vi "TestConfig.vi"(8 "error in":errorcluster {"code" format="Error %.0f"}, 11 "MainFGV_data":T1) -> (0 "error out":errorcluster {"code" format="Error %.0f"}, 3 "MainFGV_data out":T1)   [LabVIEW 2016]
uses:
  StrainGauge/SG_data.ctl
  CurrentMeter/CM_data.ctl
  CurrentMeter/CM_SerialNumber.ctl
  MainFGV_data.ctl
  Log/log_mods.ctl
  Log/log_status.ctl
panel:
  in  "OK":bool
  in  "Cancelar":bool
  in  "OpenConfig":bool caption="Abrir\nconfiguração"
  in  "SaveConfig":bool caption="Salvar\nconfiguração"
  in  "CM_config":T2[](array[typedef])=[{"Serial"=enum."274124", "Coordenada X"=0.0, "Coordenada Y"=0.0, "ID"="CH 1", "active"=TRUE}, {"Serial"=enum."274125", "Coordenada X"=0.0, "Coordenada Y"=0.0, "ID"="CH 2", "active"=TRUE}, {"Serial"=enum."274126", "Coordenada X"=0.0, "Coordenada Y"=0.0, "ID"="CH 3", "active"=TRUE}, {"Serial"=enum."274127", "Coordenada X"=0.0, "Coordenada Y"=0.0, "ID"="CH 4", "active"=TRUE}, {"Serial"=enum."274128", "Coordenada X"=0.0, "Coordenada Y"=0.0, "ID"="CH 5", "active"=TRUE}]
  in  "SG_config":T4[](array[typedef])=[{"ID"="CH 1", "Sensibilidade"=2.0, "Descrição"="Extensômetro na grade", "active"=TRUE}, {"ID"="CH 2", "Sensibilidade"=2.0, "Descrição"="Extensômetro na grade", "active"=TRUE}, {"ID"="CH 3", "Sensibilidade"=2.0, "Descrição"="Extensômetro na grade", "active"=TRUE}, {"ID"="CH 4", "Sensibilidade"=2.0, "Descrição"="Extensômetro na grade", "active"=TRUE}, {"ID"="CH 5", "Sensibilidade"=2.0, "Descrição"="Extensômetro na grade", "active"=TRUE}, {"ID"="CH 6", "Sensibilidade"=2.0, "Descrição"="Extensômetro na grade", "active"=TRUE}, {"ID"="CH 7", "Sensibilidade"=2.0, "Descrição"="Extensômetro na grade", "active"=TRUE}, {"ID"="CH 8", "Sensibilidade"=2.0, "Descrição"="Extensômetro na grade", "active"=TRUE}, {"ID"="CH 9", "Sensibilidade"=2.0, "Descrição"="Extensômetro na grade", "active"=TRUE}, {"ID"="CH 10", "Sensibilidade"=2.0, "Descrição"="Extensômetro na grade", "active"=TRUE}, {"ID"="CH 11", "Sensibilidade"=2.0, "Descrição"="Extensômetro na grade", "active"=TRUE}, {"ID"="CH 12", "Sensibilidade"=2.0, "Descrição"="Extensômetro na grade", "active"=TRUE}, {"ID"="CH 13", "Sensibilidade"=2.0, "Descrição"="Extensômetro na grade", "active"=TRUE}, {"ID"="CH 14", "Sensibilidade"=2.0, "Descrição"="Extensômetro na grade", "active"=TRUE}, {"ID"="CH 15", "Sensibilidade"=2.0, "Descrição"="Extensômetro na grade", "active"=TRUE}, {"ID"="CH 16", "Sensibilidade"=2.0, "Descrição"="Extensômetro na grade", "active"=TRUE}, {"ID"="CH 17", "Sensibilidade"=2.0, "Descrição"="Extensômetro na grade", "active"=TRUE}, {"ID"="CH 18", "Sensibilidade"=2.0, "Descrição"="Extensômetro na grade", "active"=TRUE}, {"ID"="CH 19", "Sensibilidade"=2.0, "Descrição"="Extensômetro na grade", "active"=TRUE}, {"ID"="CH 20", "Sensibilidade"=2.0, "Descrição"="Extensômetro na grade", "active"=TRUE}, {"ID"="CH 21", "Sensibilidade"=2.0, "Descrição"="Extensômetro na grade", "active"=TRUE}, {"ID"="CH 22", "Sensibilidade"=2.0, "Descrição"="Extensômetro na grade", "active"=TRUE}, {"ID"="CH 23", "Sensibilidade"=2.0, "Descrição"="Extensômetro na grade", "active"=TRUE}, {"ID"="CH 24", "Sensibilidade"=2.0, "Descrição"="Extensômetro na grade", "active"=TRUE}]
  # "Extensômetros"
  # "Molinetes"
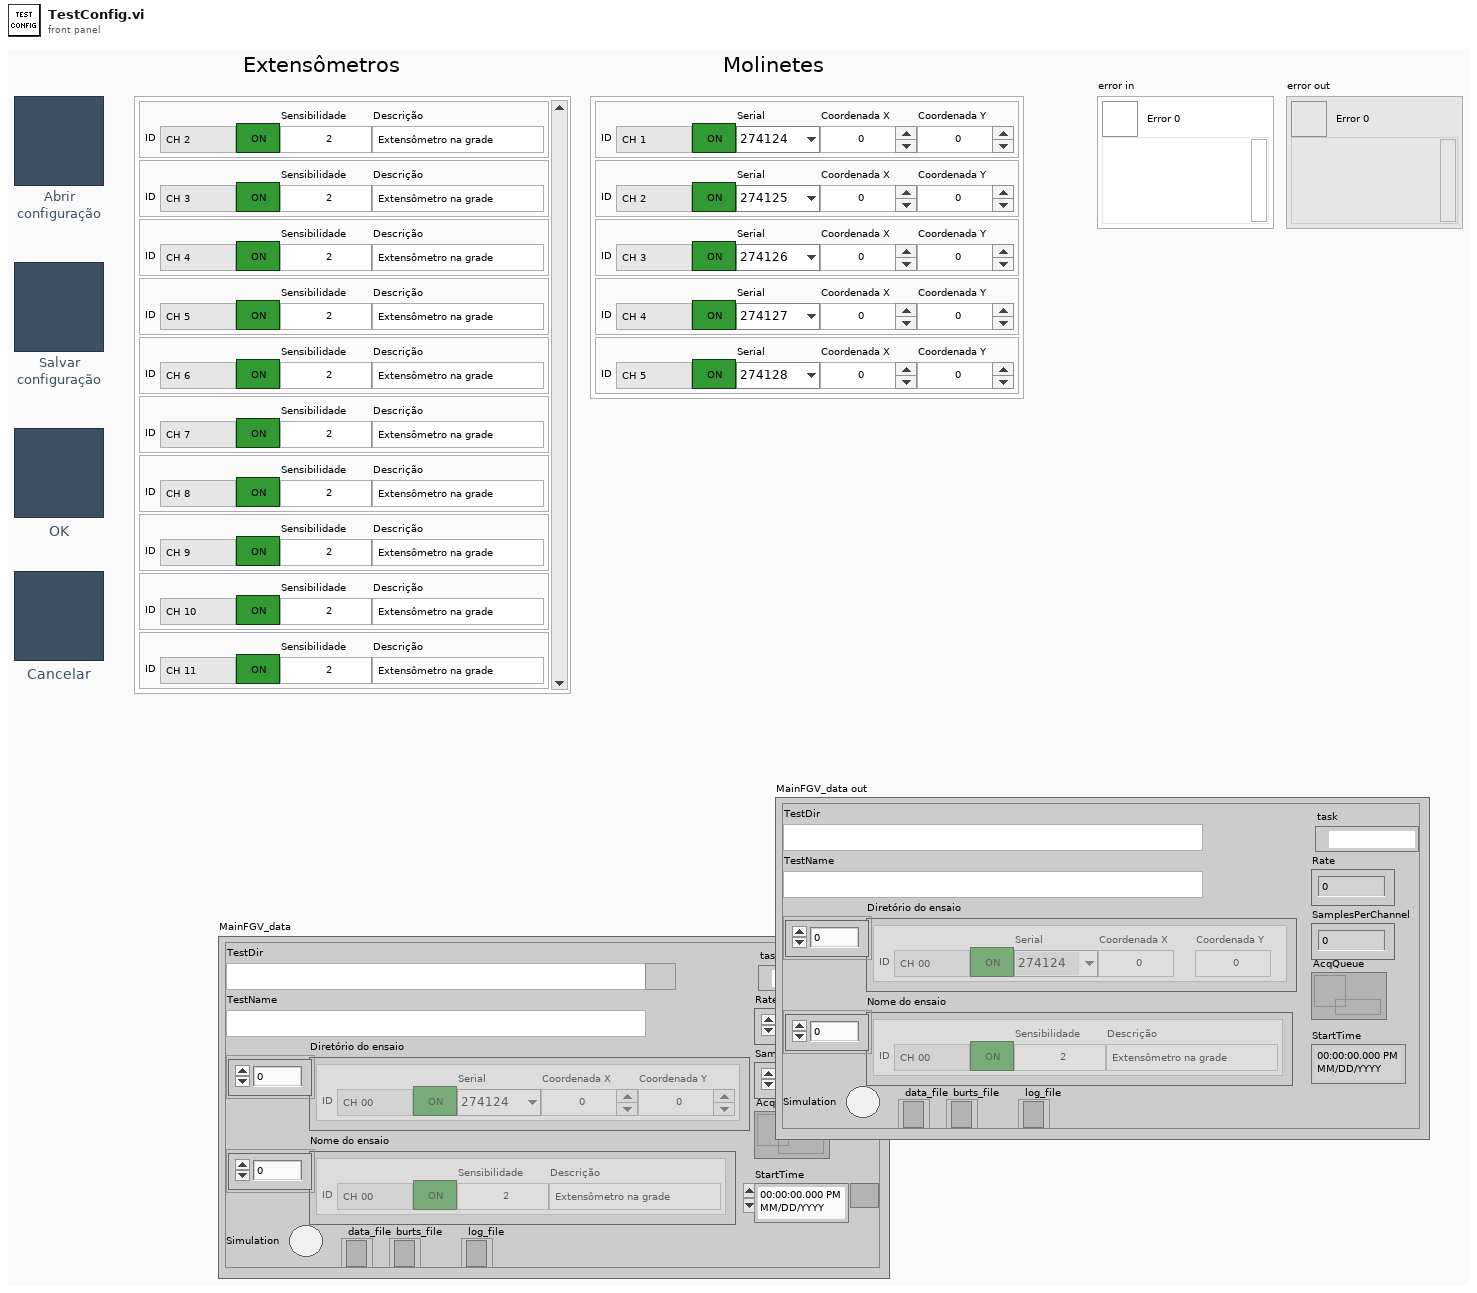
[diagram p1: front panel]
types:
  T1 = typedef "MainFGV_data.ctl" = cluster{"TestDir":path, "TestName":string, "CM_data":T2[], "SG_data":T4[], "Simulation":bool, "task":refnum<k21>, "data_file":refnum<file>, "burts_file":refnum<file>, "log_file":refnum<file>, "Rate":dbl, "SamplesPerChannel":dbl, "AcqQueue":refnum<queue>, "StartTime":timestamp}
  T2 = typedef "CM_data.ctl" = cluster{"Serial":T3, "Coordenada X":dbl, "Coordenada Y":dbl, "ID":string, "active":bool}
  T3 = typedef "CM_SerialNumber.ctl" = enum16{"274124", "274125", "274126", "274127", "274128"}
  T4 = typedef "SG_data.ctl" = cluster{"ID":string, "Sensibilidade":dbl, "Descrição":string, "active":bool}
  T5 = typedef "log_status.ctl" = enum16{"Init", "Ready", "Running", "Error", "End"}
  T6 = typedef "log_mods.ctl" = enum16{"Init", "LogFileRefnum", "SetStatus", "WriteSG", "WriteCM", "WriteToLog", "End"}
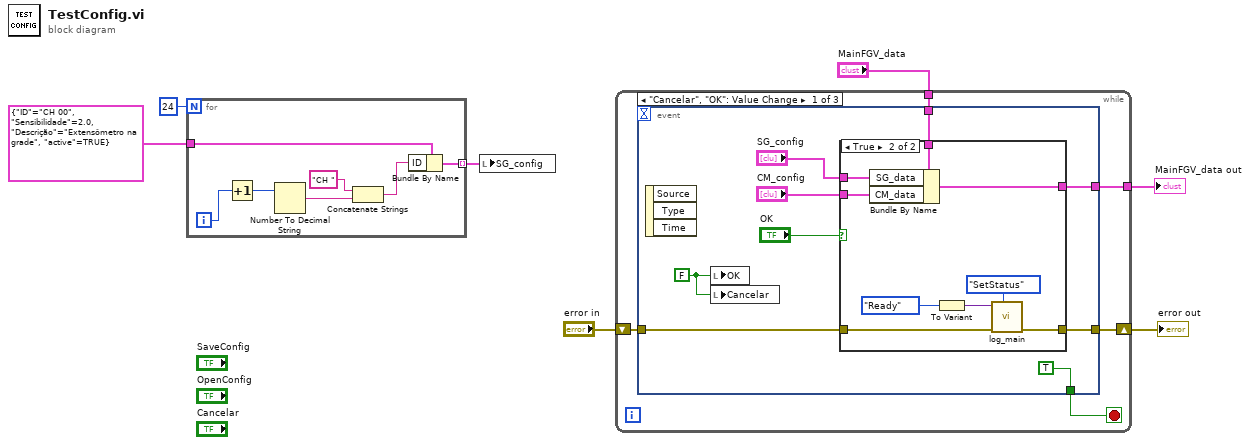
[diagram p0: block diagram]
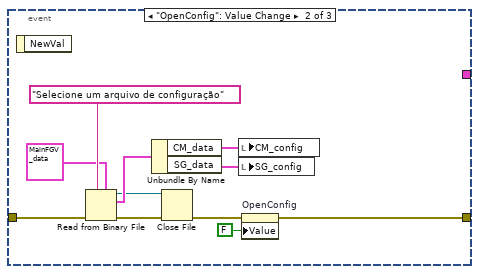
[diagram p3: hidden frame]
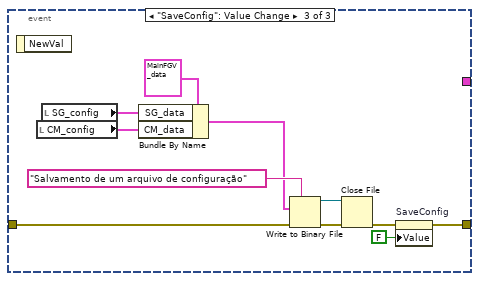
[diagram p4: hidden frame]
diagram:
  n1 = for {
    N: 24 -> [_]
    tunnel: T4 {"ID"="CH 00", "Sensibilidade"=2.0, "Descrição"="Extensômetro na grade", "active"=TRUE} ("StrainGauge_data") -> [w9]
    tunnel: [w8] -> w5 mode=indexing
    i -> [w14]
    n2 = Increment(x=w14) -> (x+1=w13:i32)
    n3 = Number To Decimal String(number=w13) -> (decimal integer string=w12:string)  [unwired: 1 in]
    n4 = Concatenate Strings("CH " ("string"), w12) -> (w10:string)
    n5 = Bundle By Name(cluster=w9, "ID"=w10) -> (w8:T4)
  }
  n6 = local write "SG_config"(w5) -> ()
  n7 = while {
    shift-right: [w17] -> w3
    shift-left: "error in" -> [w18]
    tunnel: "MainFGV_data" -> [w16]
    tunnel: [w15] -> w1
    stop <- w19 stop-if-true
    n8 = event shown="[0] \"Cancelar\", \"OK\": Value Change" {
      selector: _ -> [_ _ _]
      dyn-events: _ -> [_ _ _]
      timeout: _ -> [_ _ _]
      tunnel: [TRUE ("OK") _ _] -> w19
      tunnel: w18 -> [w21 w49 w57]
      tunnel: [w20 w40 w52] -> w17
      tunnel: w16 -> [w25 _ _]
      tunnel: [w24 _ _] -> w15
      event "Cancelar", "OK": Value Change {
        w23 = FALSE ("OK")
        n9 = event-data() -> ()  [unwired: 1 in, 3 out]
        n10 = local write "OK"(w23) -> ()
        n11 = local write "Cancelar"(w23) -> ()
        n12 = case shown="True" "OK" {
          tunnel: "CM_config" -> [_ w39]
          tunnel: "SG_config" -> [_ w38]
          tunnel: w25 -> [w30 w37]
          tunnel: [w30 w36] -> w24
          tunnel: w21 -> [w29 w32]
          tunnel: [w29 w31] -> w20
          frame False {
          }
          frame True {
            n13 = Bundle By Name(cluster=w37, "SG_data"=w38, "CM_data"=w39) -> (w36:T1)
            n14 = To Variant(anything=log_status."Ready" ("log_status")) -> (Variant=w33:variant)
            n15 = call "log_main.vi"("FGV_mods"=log_mods."SetStatus", "Error In"=w32, "DataIn"=w33) -> ("Error Out"=w31:errorcluster)  [unwired: 7 in, 1 out]
          }
        }
      }
      event "OpenConfig": Value Change {
        n16 = event-data() -> ()  [unwired: 1 in, 1 out]
        n17 = Read from Binary File(5:T1 {"TestDir"=path "C:/Users/l01481/Desktop/Teste_0", "TestName"="Teste", "CM_data"=[], "SG_data"=[], "Simulation"=TRUE, "task"="", "data_file"=refnum, "burts_file"=refnum, "log_file"=refnum, "Rate"=0.0, "SamplesPerChannel"=0.0, "AcqQueue"=refnum, "StartTime"=timestamp(0 s since 1904-01-01)} ("MainFGV_data"), 7:"Selecione um arquivo de configuração" ("prompt (Open existing file)"), 8:w49) -> (0:w46:errorcluster, 2:w47:T1, 3:w45:refnum<file>)  [unwired: 3 in, 1 out]
        n18 = Unbundle By Name(w47) -> ("CM_data"=w43:T2[], "SG_data"=w44:T4[])
        n19 = Close File(refnum=w45, error in=w46) -> (error out=w41:errorcluster)  [unwired: 1 out]
        n20 = local write "CM_config"(w43) -> ()
        n21 = local write "SG_config"(w44) -> ()
        n22 = property on="OpenConfig" class="Bool (strict)"(error in=w41, "Value"=FALSE ("SaveConfig")) -> (error out=w40:errorcluster)  [unwired: 1 in, 1 out]
      }
      event "SaveConfig": Value Change {
        n23 = event-data() -> ()  [unwired: 1 in, 1 out]
        n24 = local read "CM_config"() -> (w59:T2[])
        n25 = local read "SG_config"() -> (w60:T4[])
        n26 = Bundle By Name(cluster=T1 {"TestDir"=path "C:/Users/l01481/Desktop/Teste_0", "TestName"="Teste", "CM_data"=[], "SG_data"=[], "Simulation"=TRUE, "task"="", "data_file"=refnum, "burts_file"=refnum, "log_file"=refnum, "Rate"=0.0, "SamplesPerChannel"=0.0, "AcqQueue"=refnum, "StartTime"=timestamp(0 s since 1904-01-01)} ("MainFGV_data"), "SG_data"=w60, "CM_data"=w59) -> (w54:T1)
        n27 = Write to Binary File(data=w54, error in=w57, 7:"Salvamento de um arquivo de configuração" ("prompt (Choose or enter file path)")) -> (refnum out=w55:refnum<file>, error out=w56:errorcluster)  [unwired: 3 in, 1 out]
        n28 = Close File(refnum=w55, error in=w56) -> (error out=w53:errorcluster)  [unwired: 1 out]
        n29 = property on="SaveConfig" class="Bool (strict)"(error in=w53, "Value"=FALSE ("SaveConfig")) -> (error out=w52:errorcluster)  [unwired: 1 in, 1 out]
      }
    }
  }
  "MainFGV_data out" <- w1
  "error out" <- w3
